vi "ALINHAMENTO.vi"() -> ()   [LabVIEW 2014]
uses:
  <vilib>/Platform/TimedLoop/XDataNode/timing_clust.ctl
  <vilib>/Platform/TimedLoop/XDataNode/nitl_modes.ctl
  <vilib>/Platform/TimedLoop/XDataNode/wakeup.ctl
  <vilib>/Platform/TimedLoop/XDataNode/XDataNode.xnode
  <userlib>/Newport ESP301/Newport ESP301.lvlib
  <vilib>/Platform/TimedLoop/XDataNode/XDNodeRunTimeDep.lvlib
panel:
  in  "Home Button":bool
  out "Z Position (um)":sgl=-0.040690105 format="%#_4f"
  in  "Down Button":bool
  in  "Vertical STEP (um)":dbl=1000.0 format="%#_4g"
  in  "Up Button":bool
  in  "Zera Motor":bool
  in  "Velocity (mm/s)":sgl=0.5
  out "Motor Y\nLigado":bool=TRUE
  out "Btn Ghost":bool=TRUE
  out "X Position (mm)":dbl=1.0 format="%.6g"
  out "Y Position (mm)":dbl=-3.0 format="%.6g"
  in  "Velocity (mm/s)":dbl=10.0
  in  "Stop Button":bool
  in  "down button":bool
  in  "up button":bool
  in  "Next Button":bool
  in  "STEP (mm)":dbl=0.5
  in  "Previous Button":bool
  out "Title":string="ALIGNMENT PROCEDURE"
  # "XY PLANE"
  # "Z AXIS"
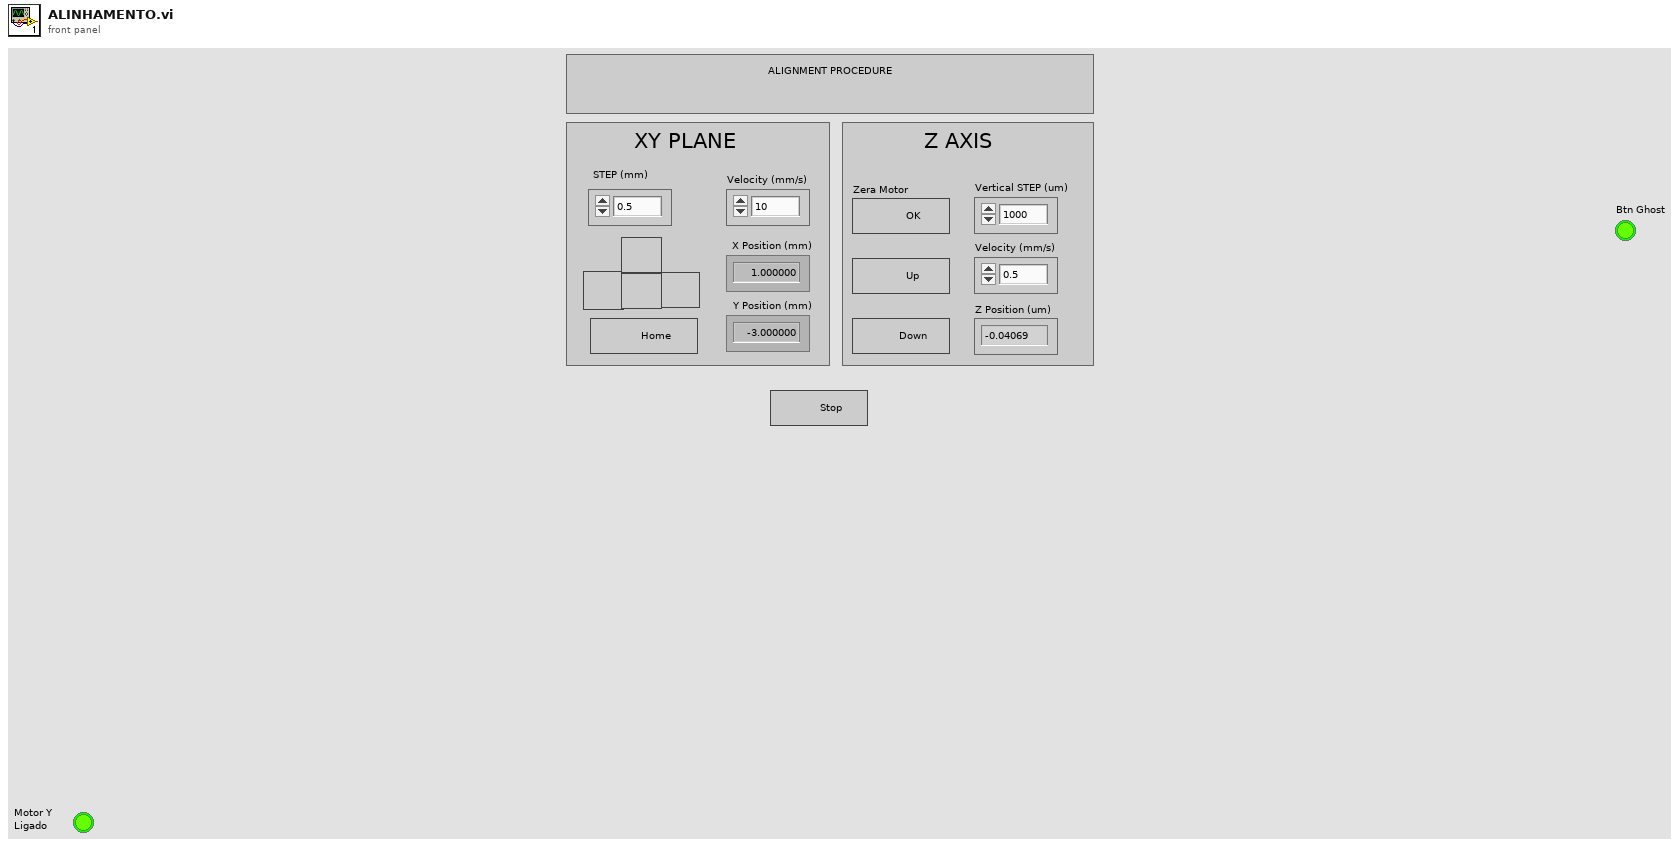
[diagram p1: front panel]
types:
  T1 = cluster{"VISA resource name":refnum<visa-resource-name>, "Device name":string, "Controller address":i32, "error":errorcluster}
  T2 = typedef "XDNodeRunTimeDep.lvlib/timing_clust.ctl" = cluster{"Expected End [f-1]":u64, "Actual End [f-1]":u64, "Finished Late? [f-1]":bool, "Expected End [i-1]":u64, "Actual End [i-1]":u64, "Finished Late? [i-1]":bool, "Expected Start [i]":u64, "Actual Start [i]":u64, "Expected Start [f]":u64, "Actual Start [f]":u64, "Source Name":string, "Structure Name":string, "Period":i64, "Deadline":i64, "Offset":i64, "Start":i64, "Priority":i32, "Timeout":i32, "Mode":T3, "Wakeup Reason":T4, "Error":errorcluster, "Source Type":string, "Secondary Source Type":string, "Global End Time":u64, "Global Start Time":u64, "Frame Duration":u64, "Iteration Duration":u64, "Assigned CPU":i32, "I/O Scan Engine Mode":u32}
  T3 = typedef "XDNodeRunTimeDep.lvlib/nitl_modes.ctl" = enum32{"No Change", "Process missed periods, maintain original phase", "Discard missed periods, maintain original phase", "Process missed periods, ignore original phase", "Discard missed periods, ignore original phase"}
  T4 = typedef "XDNodeRunTimeDep.lvlib/wakeup.ctl" = enum32{"Normal", "Aborted", "Asynchronous wakeup", "Timing source error", "Timed loop error", "Timeout"}
  T5 = enum16{"Find +0 Position Count", "Find Home and Index Signals", "Find Home Signal", "Find Positive Limit Signal", "Find Negative Limit Signal", "Find Positve Limit and Index Signals", "Find Negative Limit and Index Signals"}
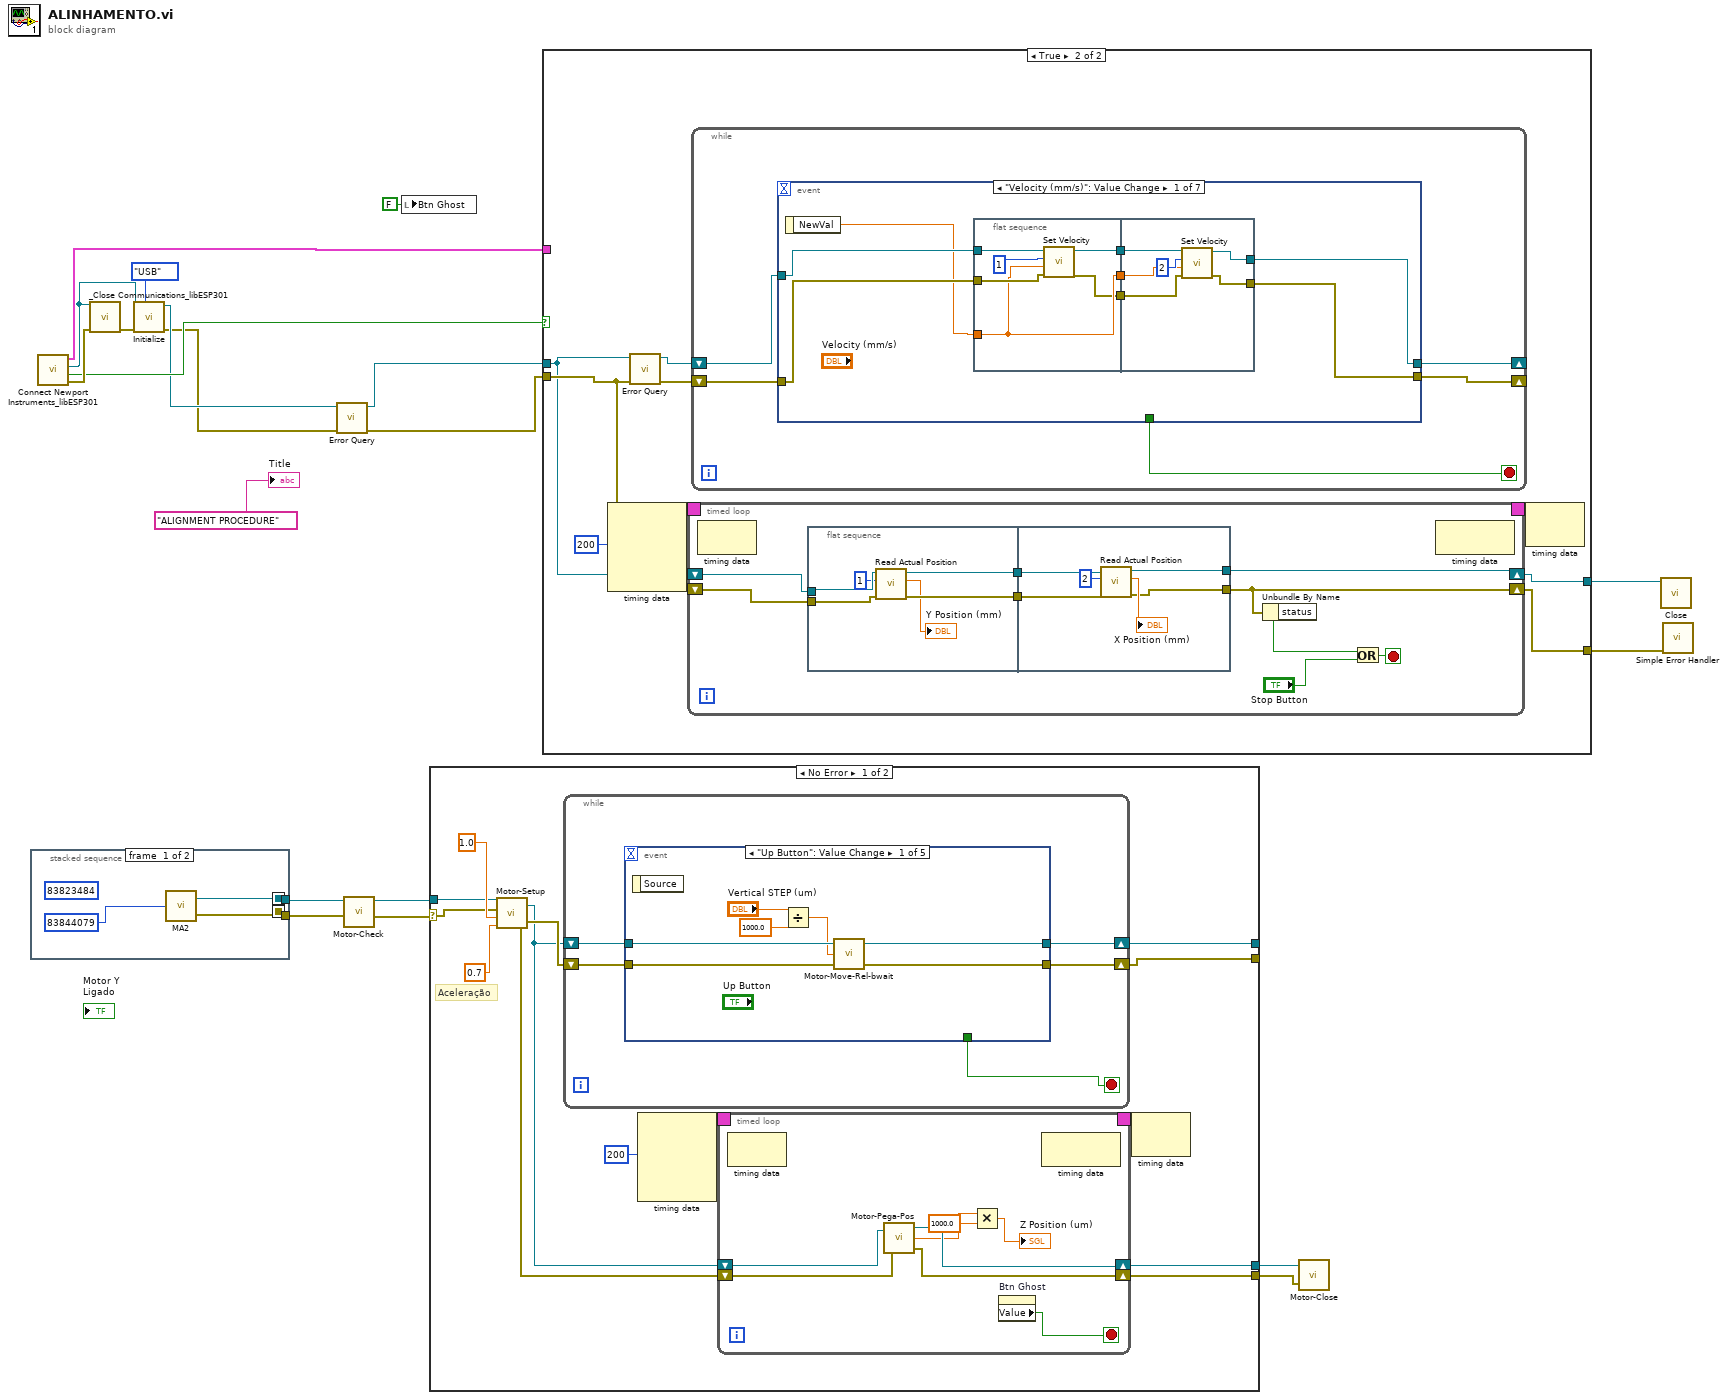
[diagram p0: block diagram]
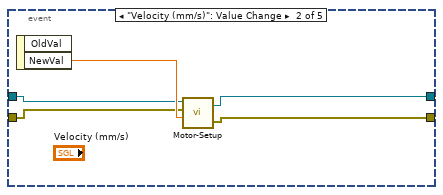
[diagram p2: hidden frame]
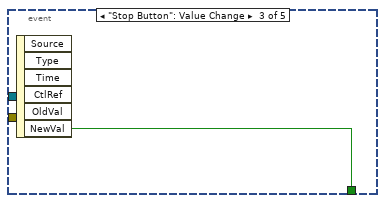
[diagram p3: hidden frame]
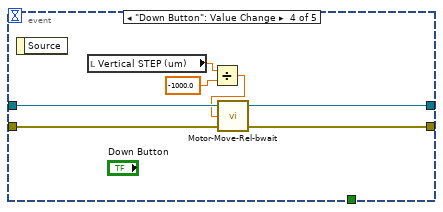
[diagram p4: hidden frame]
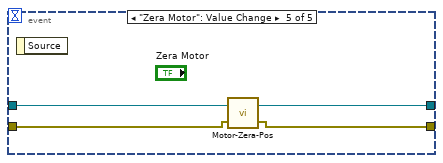
[diagram p5: hidden frame]
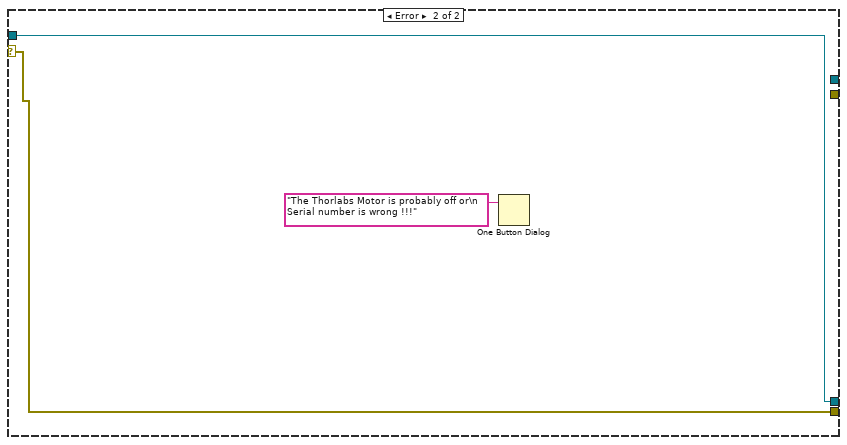
[diagram p6: hidden frame]
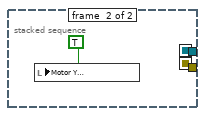
[diagram p7: hidden frame]
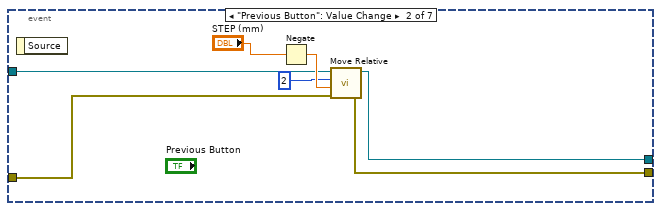
[diagram p9: hidden frame]
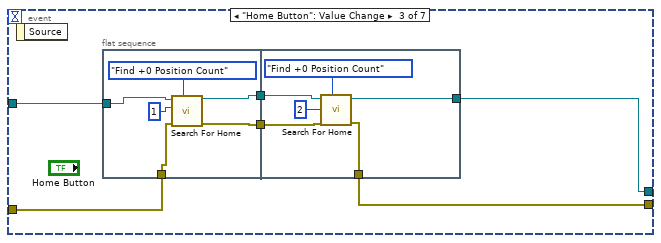
[diagram p10: hidden frame]
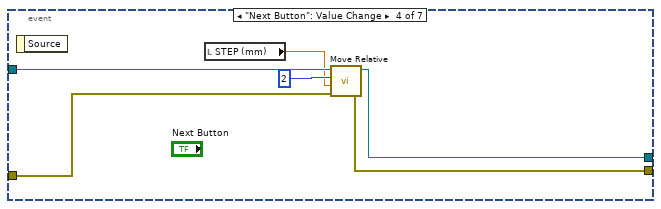
[diagram p11: hidden frame]
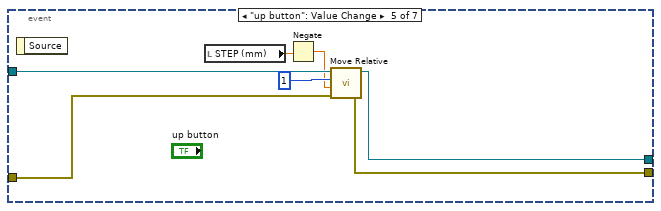
[diagram p12: hidden frame]
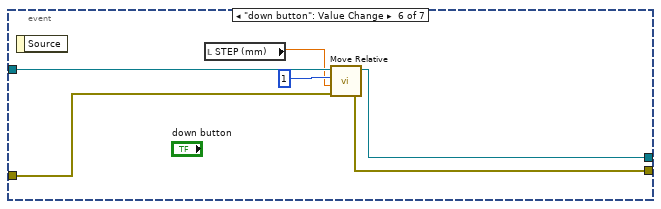
[diagram p13: hidden frame]
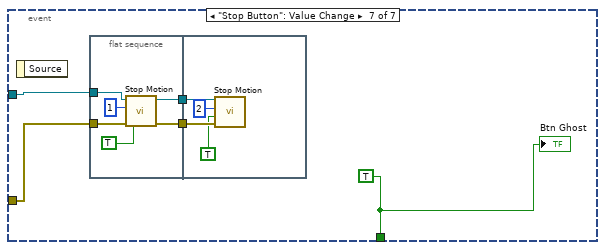
[diagram p14: hidden frame]
diagram:
  n1 = stacked-sequence {
    seq-local: [w23 _] -> [_ w26]
    seq-local: [w22 _] -> [_ w25]
    tunnel: [_ w26] -> w8
    tunnel: [_ w25] -> w5
    frame #0 {
      (unwired) 83823484 ("HWSerialNum")
      n2 = call "MA2.vi"("HWSerialNum"=83844079) -> ("MG17Motor 2"=w23:refnum<k7>, "error out"=w22:errorcluster)
    }
    frame #1 {
      n3 = local write "Motor Y\nLigado"(TRUE ("Motor3\nLigado")) -> ()
    }
  }
  n4 = call <userlib>:"Connect Newport Instruments_libESP301.vi"() -> ("error (duplicate)"=w18:errorcluster, "Connected"=w14:bool, "VISA resource name (duplicate)"=w17:refnum<visa-resource-name>, "Device Connection Cluster"=w15:T1)  [unwired: 7 in, 1 out]
  n5 = call <userlib>:"_Close Communications_libESP301.vi"("Instrument Channel"=w17, "error in (no error)"=w18) -> ("error out"=w20:errorcluster)  [unwired: 13 in]
  n6 = call <userlib>:"Initialize.vi"("VISA resource name"=w17, "error in (no error)"=w20, "Serial Link (RS232)"=enum16{"RS232", "USB"}."USB") -> ("VISA resource name out"=w4:refnum<visa-resource-name>, "error out"=w1:errorcluster)  [unwired: 6 in]
  n7 = call <userlib>:"Error Query.vi"("error in (no error)"=w1, "VISA resource name"=w4) -> ("error out"=w2:errorcluster, "VISA resource name out"=w3:refnum<visa-resource-name>)  [unwired: 2 in, 2 out]
  n8 = call "Motor-Check.vi"("error in (no error)"=w5, "Automation Refnum in"=w8) -> ("error out"=w6:errorcluster, "Automation Refnum out"=w7:refnum<k7>)  [unwired: 8 in]
  n9 = local write "Btn Ghost"(FALSE ("Boolean")) -> ()
  n10 = case shown="No Error" w6 {
    selector: w6 -> [w31 w84]
    tunnel: w7 -> [w32 w85]
    tunnel: [w30 _] -> _
    tunnel: [w29 _] -> _
    tunnel: [w28 w85] -> w10
    tunnel: [w27 w84] -> w9
    frame No Error {
      # "Aceleração"
      n11 = call "Motor-Setup.vi"("Acc"=0.7, "Velocidade"=sgl 1.0, "error"=w31, "MG17Motor A"=w32) -> ("error out"=w35:errorcluster, "MG17Motor out"=w34:refnum<k7>)
      n12 = while {
        shift-right: [w56] -> w30
        shift-left: w34 -> [w58]
        shift-right: [w55] -> w29
        shift-left: w35 -> [w57]
        stop <- w54 stop-if-true
        n13 = event shown="[0] \"Up Button\": Value Change" {
          selector: _ -> [_ _ _ _ _]
          dyn-events: _ -> [_ _ _ _ _]
          timeout: _ -> [_ _ _ _ _]
          tunnel: w58 -> [w65 w69 _ w78 w82]
          tunnel: w57 -> [w64 w68 _ w77 w81]
          tunnel: [w63 w67 _ w76 w79] -> w56
          tunnel: [w62 w66 _ w75 w80] -> w55
          tunnel: [_ _ w71 _ _] -> w54
          event "Up Button": Value Change {
            n14 = event-data() -> ()  [unwired: 1 in, 1 out]
            n15 = Divide(x="Vertical STEP (um)", y=1000.0) -> (x/y=w59:dbl)
            n16 = call "Motor-Move-Rel-bwait.vi"("error"=w64, "Posição"=w59, "MG17Motor A"=w65) -> ("error out"=w62:errorcluster, "MG17Motor out"=w63:refnum<k7>)  [unwired: 1 in]
          }
          event "Velocity (mm/s)": Value Change {
            n17 = event-data() -> ("NewVal"=w70:sgl)  [unwired: 1 in, 1 out]
            n18 = call "Motor-Setup.vi"("Velocidade"=w70, "error"=w68, "MG17Motor A"=w69) -> ("error out"=w66:errorcluster, "MG17Motor out"=w67:refnum<k7>)  [unwired: 1 in]
          }
          event "Stop Button": Value Change {
            n19 = event-data() -> ("NewVal"=w71:bool)  [unwired: 1 in, 5 out]
          }
          event "Down Button": Value Change {
            n20 = event-data() -> ()  [unwired: 1 in, 1 out]
            n21 = local read "Vertical STEP (um)"() -> (w74:dbl)
            n22 = Divide(x=w74, y=-1000.0) -> (x/y=w72:dbl)
            n23 = call "Motor-Move-Rel-bwait.vi"("error"=w77, "Posição"=w72, "MG17Motor A"=w78) -> ("error out"=w75:errorcluster, "MG17Motor out"=w76:refnum<k7>)  [unwired: 1 in]
          }
          event "Zera Motor": Value Change {
            n24 = event-data() -> ()  [unwired: 1 in, 1 out]
            n25 = call "Motor-Zera-Pos.vi"("error"=w81, "MG17Motor A"=w82) -> ("error out"=w80:errorcluster, "MG17Motor out"=w79:refnum<k7>)
          }
        }
      }
      n26 = node-c288(i64 200 ("Period")) -> (w39:T2)  [unwired: 3 in]
      n27 = timed-loop {
        timing: w39 -> [_]
        timing-out: [_] -> w38
        shift-right: [w44] -> w28
        shift-left: w34 -> [w47]
        shift-right: [w45] -> w27
        shift-left: w35 -> [w46]
        stop <- w43 stop-if-true
        n28 = node-c288() -> ()  [unwired: 1 in, 1 out]
        n29 = call "Motor-Pega-Pos.vi"("MG17Motor 2"=w47, "error out"=w46) -> ("MG17Motor 3"=w44:refnum<k7>, "pfPosition"=w41:sgl, "error out 2"=w45:errorcluster)
        n30 = Multiply(x=w41, y=sgl 1000.0) -> (x*y=→"Z Position (um)":sgl)
        n31 = property on="Btn Ghost" class="Bool (strict)"() -> ("Value"=w43:bool)  [unwired: 2 in, 2 out]
        n32 = node-c288() -> ()  [unwired: 1 in, 1 out]
      }
      n33 = node-c288(w38) -> ()  [unwired: 1 out]
    }
    frame Error {
      n34 = One Button Dialog(message="The Thorlabs Motor is probably off or\n Serial number is wrong !!!") -> ()  [unwired: 1 in, 1 out]
    }
  }
  n35 = case shown="True" w14 {
    tunnel: w15 -> [_ _]
    tunnel: w2 -> [w87 w91]
    tunnel: w3 -> [w86 w90]
    tunnel: [w86 w89] -> w13
    tunnel: [w87 w88] -> w12
    frame False {
    }
    frame True {
      n36 = node-c288(i64 200 ("Period")) -> (w94:T2)  [unwired: 3 in]
      n37 = call <userlib>:"Error Query.vi"("error in (no error)"=w91, "VISA resource name"=w90) -> ("error out"=w95:errorcluster, "VISA resource name out"=w96:refnum<visa-resource-name>)  [unwired: 2 in, 2 out]
      n38 = timed-loop {
        timing: w94 -> [_]
        timing-out: [_] -> w93
        shift-right: [w101] -> w89
        shift-left: w90 -> [w105]
        shift-right: [w100] -> w88
        shift-left: w91 -> [w104]
        stop <- w97 stop-if-true
        n39 = node-c288() -> ()  [unwired: 1 in, 1 out]
        n40 = flat-sequence {
          tunnel: w105 -> [w111]
          tunnel: w104 -> [w110]
          tunnel: [w109] -> w103
          tunnel: [w108] -> w102
          tunnel: w103 -> [w117]
          tunnel: w102 -> [w116]
          tunnel: [w113] -> w101
          tunnel: [w112] -> w100
          frame #0 {
            n41 = call <userlib>:"Read Actual Position.vi"("error in (no error)"=w110, "Axis (1)"=1, "VISA resource name"=w111) -> ("error out"=w108:errorcluster, "Position (units)"=→"Y Position (mm)":dbl, "VISA resource name out"=w109:refnum<visa-resource-name>)  [unwired: 2 in]
          }
          frame #1 {
            n42 = call <userlib>:"Read Actual Position.vi"("error in (no error)"=w116, "Axis (1)"=2, "VISA resource name"=w117) -> ("error out"=w112:errorcluster, "Position (units)"=→"X Position (mm)":dbl, "VISA resource name out"=w113:refnum<visa-resource-name>)  [unwired: 2 in]
          }
        }
        n43 = Unbundle By Name(w100) -> ("status"=w99:bool)
        n44 = Or(x=w99, y="Stop Button") -> (x .or. y?=w97:bool)
        n45 = node-c288() -> ()  [unwired: 1 in, 1 out]
      }
      n46 = while {
        shift-right: [w125] -> _
        shift-left: w95 -> [w127]
        shift-right: [w126] -> _
        shift-left: w96 -> [w128]
        stop <- w124 stop-if-true
        n47 = event shown="[0] \"Velocity (mm/s)\": Value Change" {
          selector: _ -> [_ _ _ _ _ _ _]
          dyn-events: _ -> [_ _ _ _ _ _ _]
          timeout: _ -> [_ _ _ _ _ _ _]
          tunnel: w128 -> [w135 w153 w161 w178 w185 w191 w197]
          tunnel: w127 -> [w133 w152 w160 w177 w184 w190 w196]
          tunnel: [w134 w150 w156 w175 w183 w189 _] -> w126
          tunnel: [w132 w149 w157 w174 w182 w188 _] -> w125
          tunnel: [_ _ _ _ _ _ w193] -> w124
          event "Velocity (mm/s)": Value Change {
            n48 = event-data() -> ("NewVal"=w129:dbl)  [unwired: 1 in]
            n49 = flat-sequence {
              tunnel: w129 -> [w138]
              tunnel: [w138] -> w136
              tunnel: w135 -> [w142]
              tunnel: w133 -> [w139]
              tunnel: [w141] -> w131
              tunnel: [w137] -> w130
              tunnel: w136 -> [w145]
              tunnel: [w147] -> w134
              tunnel: [w143] -> w132
              tunnel: w131 -> [w148]
              tunnel: w130 -> [w144]
              frame #0 {
                n50 = call <userlib>:"Set Velocity.vi"("error in (no error)"=w139, "Velocity (units/s)"=w138, "Axis (1)"=1, "VISA resource name"=w142) -> ("error out"=w137:errorcluster, "VISA resource name out"=w141:refnum<visa-resource-name>)  [unwired: 2 in]
              }
              frame #1 {
                n51 = call <userlib>:"Set Velocity.vi"("error in (no error)"=w144, "Velocity (units/s)"=w145, "Axis (1)"=2, "VISA resource name"=w148) -> ("error out"=w143:errorcluster, "VISA resource name out"=w147:refnum<visa-resource-name>)  [unwired: 2 in]
              }
            }
          }
          event "Previous Button": Value Change {
            n52 = event-data() -> ()  [unwired: 1 in, 1 out]
            n53 = Negate(x="STEP (mm)") -> (-x=w155:dbl)
            n54 = call <userlib>:"Move Relative.vi"("error in (no error)"=w152, "Position (0 units)"=w155, "Axis (1)"=2, "VISA resource name"=w153) -> ("error out"=w149:errorcluster, "VISA resource name out"=w150:refnum<visa-resource-name>)  [unwired: 2 in]
          }
          event "Home Button": Value Change {
            n55 = event-data() -> ()  [unwired: 1 in, 1 out]
            n56 = flat-sequence {
              tunnel: w161 -> [w167]
              tunnel: w160 -> [w166]
              tunnel: [w163] -> w159
              tunnel: [w162] -> w158
              tunnel: w159 -> [w171]
              tunnel: w158 -> [w170]
              tunnel: [w169] -> w157
              tunnel: [w168] -> w156
              frame #0 {
                n57 = call <userlib>:"Search For Home.vi"("Home mode"=T5."Find +0 Position Count", "error in (no error)"=w166, "Axis (1)"=1, "VISA resource name"=w167) -> ("error out"=w162:errorcluster, "VISA resource name out"=w163:refnum<visa-resource-name>)  [unwired: 3 in]
              }
              frame #1 {
                n58 = call <userlib>:"Search For Home.vi"("Home mode"=T5."Find +0 Position Count", "error in (no error)"=w170, "Axis (1)"=2, "VISA resource name"=w171) -> ("error out"=w169:errorcluster, "VISA resource name out"=w168:refnum<visa-resource-name>)  [unwired: 3 in]
              }
            }
          }
          event "Next Button": Value Change {
            n59 = event-data() -> ()  [unwired: 1 in, 1 out]
            n60 = local read "STEP (mm)"() -> (w176:dbl)
            n61 = call <userlib>:"Move Relative.vi"("error in (no error)"=w177, "Position (0 units)"=w176, "Axis (1)"=2, "VISA resource name"=w178) -> ("error out"=w174:errorcluster, "VISA resource name out"=w175:refnum<visa-resource-name>)  [unwired: 2 in]
          }
          event "up button": Value Change {
            n62 = event-data() -> ()  [unwired: 1 in, 1 out]
            n63 = local read "STEP (mm)"() -> (w181:dbl)
            n64 = Negate(x=w181) -> (-x=w180:dbl)
            n65 = call <userlib>:"Move Relative.vi"("error in (no error)"=w184, "Position (0 units)"=w180, "Axis (1)"=1, "VISA resource name"=w185) -> ("error out"=w182:errorcluster, "VISA resource name out"=w183:refnum<visa-resource-name>)  [unwired: 2 in]
          }
          event "down button": Value Change {
            n66 = event-data() -> ()  [unwired: 1 in, 1 out]
            n67 = local read "STEP (mm)"() -> (w187:dbl)
            n68 = call <userlib>:"Move Relative.vi"("error in (no error)"=w190, "Position (0 units)"=w187, "Axis (1)"=1, "VISA resource name"=w191) -> ("error out"=w188:errorcluster, "VISA resource name out"=w189:refnum<visa-resource-name>)  [unwired: 2 in]
          }
          event "Stop Button": Value Change {
            w193 = TRUE ("Stop all axes (F)")
            n69 = event-data() -> ()  [unwired: 1 in, 1 out]
            n70 = flat-sequence {
              tunnel: w197 -> [w203]
              tunnel: w196 -> [w202]
              tunnel: [w200] -> w195
              tunnel: [w199] -> w194
              tunnel: w195 -> [w207]
              tunnel: w194 -> [w206]
              frame #0 {
                n71 = call <userlib>:"Stop Motion.vi"("error in (no error)"=w202, "Stop all axes (F)"=TRUE, "Axis (1)"=1, "VISA resource name"=w203) -> ("error out"=w199:errorcluster, "VISA resource name out"=w200:refnum<visa-resource-name>)  [unwired: 2 in]
              }
              frame #1 {
                n72 = call <userlib>:"Stop Motion.vi"("error in (no error)"=w206, "Stop all axes (F)"=TRUE, "Axis (1)"=2, "VISA resource name"=w207) -> ()  [unwired: 2 in, 2 out]
              }
            }
            "Btn Ghost" <- w193
          }
        }
      }
      n73 = node-c288(w93) -> ()  [unwired: 1 out]
    }
  }
  n74 = call "Motor-Close.vi"("error out"=w9, "MG17Motor 3"=w10) -> ()  [unwired: 1 in]
  n75 = call <userlib>:"Close.vi"("VISA resource name"=w13) -> ()  [unwired: 10 in, 1 out]
  n76 = call <vilib>:"Simple Error Handler.vi"("error in (no error)"=w12) -> ()  [unwired: 1 in, 8 out]
  "Title" <- "ALIGNMENT PROCEDURE" ("Title")
